vi "Get Devices List.vi"(0 "SLSC Remote in":refnum<class "SLSC Remote.lvclass">, 11 "error in (no error)":errorcluster) -> (4 "SLSC Remote out":refnum<class "SLSC Remote.lvclass">, 8 "Sys.Devices":refnum<k21>[](array[refnum]), 15 "error out":errorcluster)   [LabVIEW 2016, in "SLSC Interfaces.lvlib" / "SLSC Remote.lvclass"]
uses:
  SLSC Remote.lvclass
  C:/Users/tblair/Documents/SLSC-Interface/Source/SLSC Interface Class/SLSC Interface.lvclass
  <vilib>/rajsite/i3-json/JSON Generation/Create Value Files/Create Value - Object.vi
  <vilib>/rajsite/i3-json/JSON Generation/Add Object Parameter Files/Add Object Parameter - String.vi
  <vilib>/NI/NI JSONRPC Server Framework/Classes/Server/Format Client Request (Auto-Increment).vi
  <vilib>/httpClient/POSTBuffer.vi
  <vilib>/rajsite/i3-json/JSON Parsing/Get Object Parameter Files/Get Object Parameter - 1D Array String.vi
  <vilib>/NI/NI JSONRPC Server Framework/Classes/Server/JSONRPC Server.lvclass
  <vilib>/rajsite/i3-json/i3-json.lvlib
  <vilib>/httpClient/LabVIEWHTTPClient.lvlib
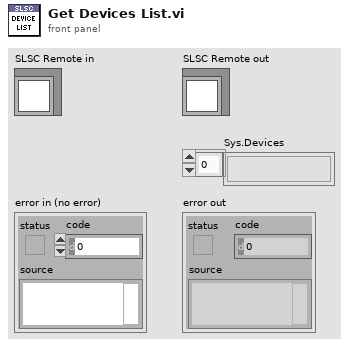
[diagram p1: front panel]
types:
  T1 = typedef "LabVIEWHTTPClient.lvlib/ClientHandle.ctl" = refnum<k1>
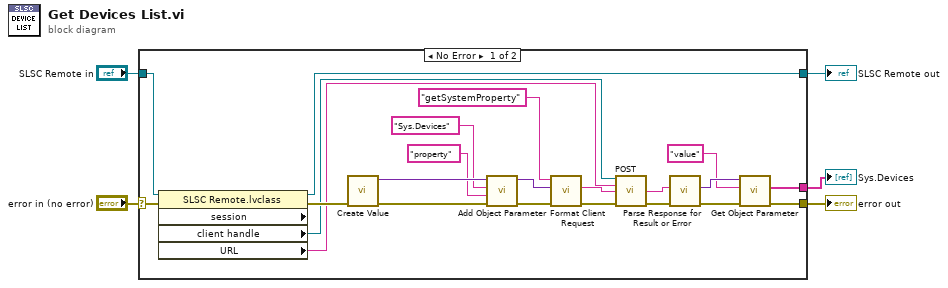
[diagram p0: block diagram]
diagram:
  n1 = case shown="No Error" "error in (no error)" {
    selector: "error in (no error)" -> [w24 w28]
    tunnel: "SLSC Remote in" -> [w26 w29]
    tunnel: [w25 w29] -> w3
    tunnel: [w12 w28] -> w1
    tunnel: [w11 _] -> w2
    frame No Error {
      n2 = property class="SLSC Remote.lvclass" props=["session", "client handle", "URL"](reference=w26, error in=w24) -> (reference out=w25:refnum<class "SLSC Remote.lvclass">, error out=w23:errorcluster, "client handle"=w19:T1, "URL"=w18:string)  [unwired: 1 out]
      n3 = call-poly <vilib>:"Create Value.vi"("error in (no error)"=w23) -> ("error out"=w22:errorcluster, "JSON Tree"=w27:variant)  [unwired: 9 in]
      n4 = call-poly <vilib>:"Add Object Parameter.vi"("error in (no error)"=w22, "Name"="property", "String"="Sys.Devices", "JSON Tree in (JSON Object)"=w27) -> ("error out"=w8:errorcluster, "JSON Tree out (JSON Object)"=w9:variant)  [unwired: 6 in]
      n5 = call-poly <vilib>:"Format Client Request.vi"("error in (no error)"=w8, "params"=w9, "method"="getSystemProperty") -> ("error out"=w17:errorcluster, "Request String"=w20:string)  [unwired: 7 in]
      n6 = call-poly <vilib>:"POST.vi"("client handle"=w19, "url"=w18, "buffer"=w20, "error in (no error)"=w17) -> ("body"=w16:string, "error out"=w15:errorcluster)  [unwired: 8 in, 2 out]
      n7 = call <vilib>:"Parse Response for Result or Error.vi"("error in"=w15, "Response String In"=w16) -> ("error out"=w13:errorcluster, "Result or Error Data"=w14:variant)  [unwired: 7 in, 1 out]
      n8 = call-poly <vilib>:"Get Object Parameter.vi"("error in (no error)"=w13, "Parameter Name"="value", "JSON Tree In (JSON Object)"=w14) -> ("error out"=w12:errorcluster, "1D String Array Value"=w11:string[])  [unwired: 5 in, 2 out]
    }
    frame Error {
    }
  }
  "error out" <- w1
  "SLSC Remote out" <- w3
  "Sys.Devices" <- w2
